vi "Main.vi"() -> ()   [LabVIEW 2015]
panel:
  out "input 2":dbl[](array[numeric])
  in  "input":dbl[](array[numeric])
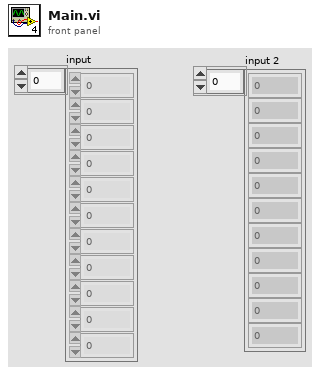
[diagram p1: front panel]
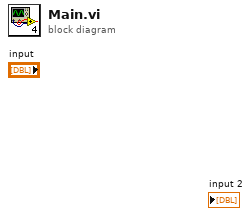
[diagram p0: block diagram]
diagram:
